vi "保存文件.vi"(8 "input":string, 9 "名称或相对路径":string="output", 10 "路径 input":path, 11 "文件名":string="config.json") -> (2 "output":string)   [LabVIEW 2019]
panel:
  out "路径":string
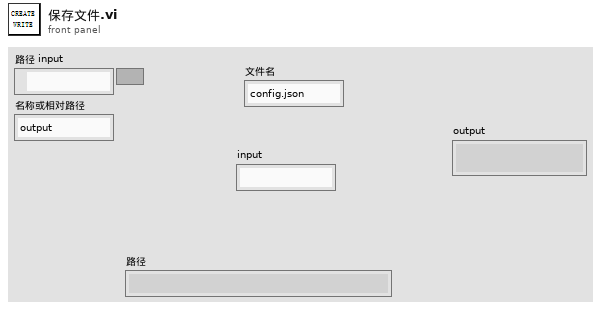
[diagram p1: front panel]
types:
  T1 = enum16{"open", "replace", "create", "open or create", "replace or create", "replace or create with confirmation"}
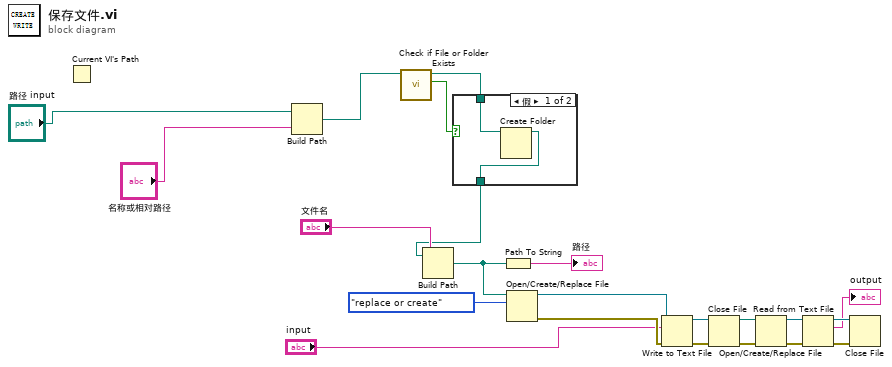
[diagram p0: block diagram]
diagram:
  n1 = Current VI's Path() -> ()  [unwired: 1 out]
  n2 = Build Path(base path="路径 input", name or relative path="名称或相对路径") -> (appended path=w6:path)
  n3 = call <vilib>:"Check if File or Folder Exists.vi"("path"=w6) -> ("file or folder exists?"=w5:bool, "dup path"=w4:path)  [unwired: 8 in, 1 out]
  n4 = case shown="假" w5 {
    tunnel: w4 -> [w24 w25]
    tunnel: [w23 w25] -> w3
    frame False {
      n5 = Create Folder(path (use dialog)=w24) -> (created path=w23:path)  [unwired: 2 in, 2 out]
    }
    frame True {
    }
  }
  n6 = Build Path(base path=w3, name or relative path="文件名") -> (appended path=w19:path)
  n7 = Path To String(path=w19) -> (string=→"路径":string)
  n8 = Open/Create/Replace File(file path (use dialog)=w19, operation (0:open)=T1."replace or create" ("操作(0:open)")) -> (refnum out=w20:refnum<file>, error out=w21:errorcluster)  [unwired: 4 in, 1 out]
  n9 = Write to Text File(file (use dialog)=w20, text="input", error in=w21) -> (refnum out=w17:refnum<file>, error out=w16:errorcluster)  [unwired: 1 in, 1 out]
  n10 = Close File(refnum=w17, error in=w16) -> (path=w15:path, error out=w14:errorcluster)
  n11 = Open/Create/Replace File(file path (use dialog)=w15, error in=w14) -> (refnum out=w13:refnum<file>, error out=w12:errorcluster)  [unwired: 4 in, 1 out]
  n12 = Read from Text File(file (use dialog)=w13, error in=w12) -> (refnum out=w11:refnum<file>, text=→"output":string, error out=w10:errorcluster)  [unwired: 2 in, 1 out]
  n13 = Close File(refnum=w11, error in=w10) -> ()  [unwired: 2 out]
